vi "Attack.vi"(6 "Direction":T1, 7 "Next Play":u32, 9 "YX Type":string, 11 "Maze 2.0.lvclass":refnum<class "Maze 2.0.lvclass">) -> (1 "Success?":bool)   [LabVIEW 2014, in "Maze 2.0.lvclass"]
uses:
  Maze 2.0.lvclass
  Direction Enum.ctl
  Maze 2.0.lvclass/Maze 2.0.ctl
  Runner Cluster.ctl
  Runner/Runner.lvclass
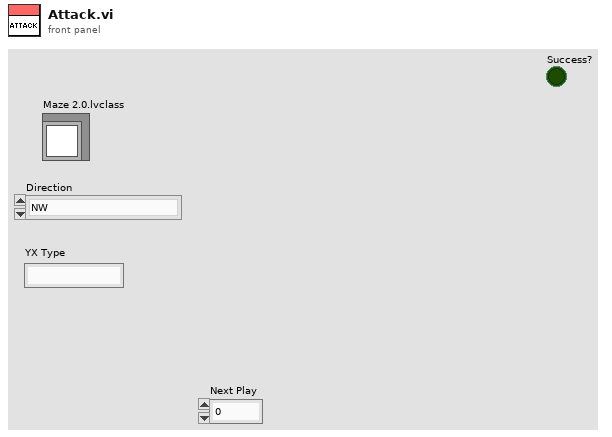
[diagram p1: front panel]
types:
  T1 = typedef "Maze 2.0.lvclass/Direction Enum.ctl" = enum16{"NW", "N", "NE", "E", "SE", "S", "SW", "W"}
  T2 = typedef "Maze 2.0.lvclass/Runner Cluster.ctl" = cluster{"Alive?":bool, "RunnerRef":refnum<data-value>, "TeamIdx":i32, "Player #":i32, "NextPlay":u32}
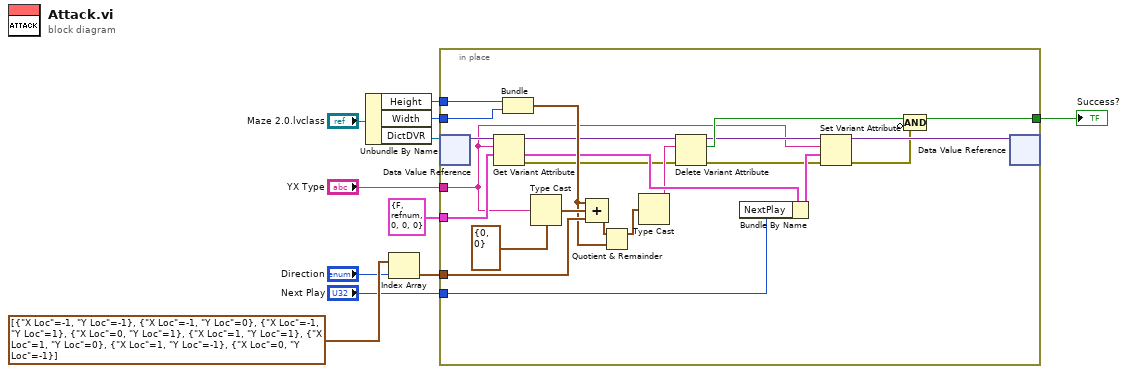
[diagram p0: block diagram]
diagram:
  n1 = Unbundle By Name("Maze 2.0.lvclass") -> ("Height"=w4:i32, "Width"=w3:i32, "DictDVR"=w5:refnum<data-value>)
  n2 = Index Array(array=cluster{"X Loc":i32, "Y Loc":i32}[] [{"X Loc"=-1, "Y Loc"=-1}, {"X Loc"=-1, "Y Loc"=0}, {"X Loc"=-1, "Y Loc"=1}, {"X Loc"=0, "Y Loc"=1}, {"X Loc"=1, "Y Loc"=1}, {"X Loc"=1, "Y Loc"=0}, {"X Loc"=1, "Y Loc"=-1}, {"X Loc"=0, "Y Loc"=-1}], index="Direction") -> (element=w7:cluster{"X Loc":i32, "Y Loc":i32})
  n3 = in-place {
    in-place-border: "YX Type" -> [w15]
    in-place-border: T2 {"Alive?"=FALSE, "RunnerRef"=refnum, "TeamIdx"=0, "Player #"=0, "NextPlay"=0} ("Cluster") -> [w33]
    in-place-border: w7 -> [w28]
    in-place-border: w4 -> [w32]
    in-place-border: w3 -> [w31]
    in-place-border: [w13] -> w2
    in-place-border: "Next Play" -> [w23]
    n4 = in-place-dvr #1(w5) -> (w34:variant)  [unwired: 1 out]
    n5 = Get Variant Attribute(Variant=w34, name=w15, default value (empty Variant)=w33) -> (duplicate Variant=w21:variant, value=w24:T2, error out=w20:errorcluster)  [unwired: 1 in, 1 out]
    n6 = Bundle("Height"=w32, "Width"=w31) -> (w26:cluster{"Height":i32, "Width":i32})  [unwired: 1 in]
    n7 = Type Cast(type=cluster{"Y":i32, "X":i32} {"Y"=0, "X"=0}, x=w15) -> (*(type *) &x=w27:cluster{"Y":i32, "X":i32})
    n8 = Compound Arithmetic op=ADD(w26, w27, w28) -> (w30:cluster{i32, i32})
    n9 = Quotient & Remainder(x=w30, y=w26) -> (x-y*floor(x/y)=w25:cluster{i32, i32})  [unwired: 1 out]
    n10 = Type Cast(x=w25) -> (*(type *) &x=w22:string)  [unwired: 1 in]
    n11 = Delete Variant Attribute(4:w20, 6:w22, 7:w21) -> (0:w16:errorcluster, 2:w19:bool, 3:w17:variant)
    n12 = Bundle By Name(cluster=w24, "NextPlay"=w23) -> (w18:T2)
    n13 = Set Variant Attribute(Variant=w17, name=w15, value=w18, error in=w16) -> (Variant out=w14:variant, error out=w12:errorcluster)  [unwired: 1 out]
    n14 = Compound Arithmetic op=AND(w19, invert w12) -> (w13:bool)
    n15 = in-place-dvr #1(w14) -> ()  [unwired: 2 out]
  }
  "Success?" <- w2
